vi "GlueRepeatedLinePattern.vi"(2 "Controller In":refnum<k24>, 3 "Dry Run":bool, 5 "Module Number":i32=7, 6 "Calibration Directory":path) -> (0 ".NET Refnum out":refnum<k24>)   [LabVIEW 2016]
uses:
  <vilib>/LabVIEW Interface for Arduino/Type Defs/Arduino Resource.ctl
  <vilib>/LabVIEW Interface for Arduino/Type Defs/Board Type.ctl
  C:/Users/Aerotech/Documents/BNLStaveAssembly-blueprint/Bin/Aerotech.A3200.dll
  BNLStaveAssembly-blueprint/Bin/Aerotech.A3200.dll
  <vilib>/LabVIEW Interface for Arduino/Type Defs/Pin Mode.ctl
  <vilib>/Utility/file.llb/Read Delimited Spreadsheet (DBL).vi
  <vilib>/LabVIEW Interface for Arduino/LabVIEW Interface for Arduino.lvlib
panel:
  out "Line Motion":T1
  out "Finished":bool
  out "N Lines":i32
  out "Lines Glued":i32
  out "Elapsed Time [s]":dbl format="%.2g"
  out "Shift to Start [mm]":dbl[](array[numeric]) format="%.1f"
  out "Start Position [mm]":dbl[](array[numeric]) format="%#.3g"
  in  "Abort stage":bool
  in  "Pattern Indicator":enum32{"Glue Pattern"}(tab)
  out "Relative Line\nSeparations [mm]":dbl[][](array[numeric])=[[18.5, 7.25], [2.5, 3.5], [-3.5, 5.0], [2.5, 3.15], [2.5, 3.15], [2.5, 3.15], [2.5, 3.15], [2.5, 3.15], [2.5, 3.15], [2.5, 3.15], [2.5, 3.15], [2.5, 3.15], [2.5, 3.15], [2.5, 3.15], [3.75, 5.0], [2.5, 3.5]] format="%#_13g"
  out "Line Lengths [mm]":dbl[](array[numeric])=[65.0, 65.0, 73.5, 73.5, 73.5, 73.5, 73.5, 73.5, 73.5, 73.5, 73.5, 73.5, 73.5, 73.5, 65.0, 65.0] format="%#_13g"
  out "Motion Time [s]":dbl[](array[numeric])
  in  "Outputs Tab":enum32{"Running Positions"}(tab)
  out "Running Positions [mm]":dbl[][](array[numeric])
  in  "Times [s]":dbl[](array[numeric])
  out "Running Times [s]":dbl[](array[numeric])
  in  "Inputs Tab":T2(tab)
  out "Virtual Stave Map":path
  out "Stave Angle [rad]":dbl format="%#_13g"
  out "Stereo Angle [mrad]":dbl=-26.0 format="%#_13g"
  out "Total Angle [rad]":dbl
  out "Orientation":string
  out "Pin Down?":bool
  in  "Pulse Length [ms]":dbl=125.0 format="%#_13g"
  out "Arduino Resource":T3={"VISA resource"="GlueCTRL", "Board Type"=enum."Uno", "Connection Type"=enum."USB / Serial", "Bytes Per Packet (15)"=15}
  in  "Digital I/O Pin":u8=7
  in  "Default Axis Speeds":T5={"X [mm/s]"=25.0, "Y [mm/s]"=25.0, "Z [mm/s]"=25.0}
  in  "Camera to Dispenser \nShift [mm]":dbl[](array[numeric])=[107.938, 5.003, 0.0]
  in  "Glue Pattern .csv File":path=path "C:/Users/Aerotech/Documents/BNL_ThermomechanicalStave/1_ModulePlacement/1_GluePatterning/Glue/GluePatterns/Pattern9-8.txt"
  in  "Axial":bool
  in  "Wait [ms]":dbl=750.0 format="%#_13g"
  in  "Positions [mm]":dbl[][](array[numeric])
  in  "Terminate":bool
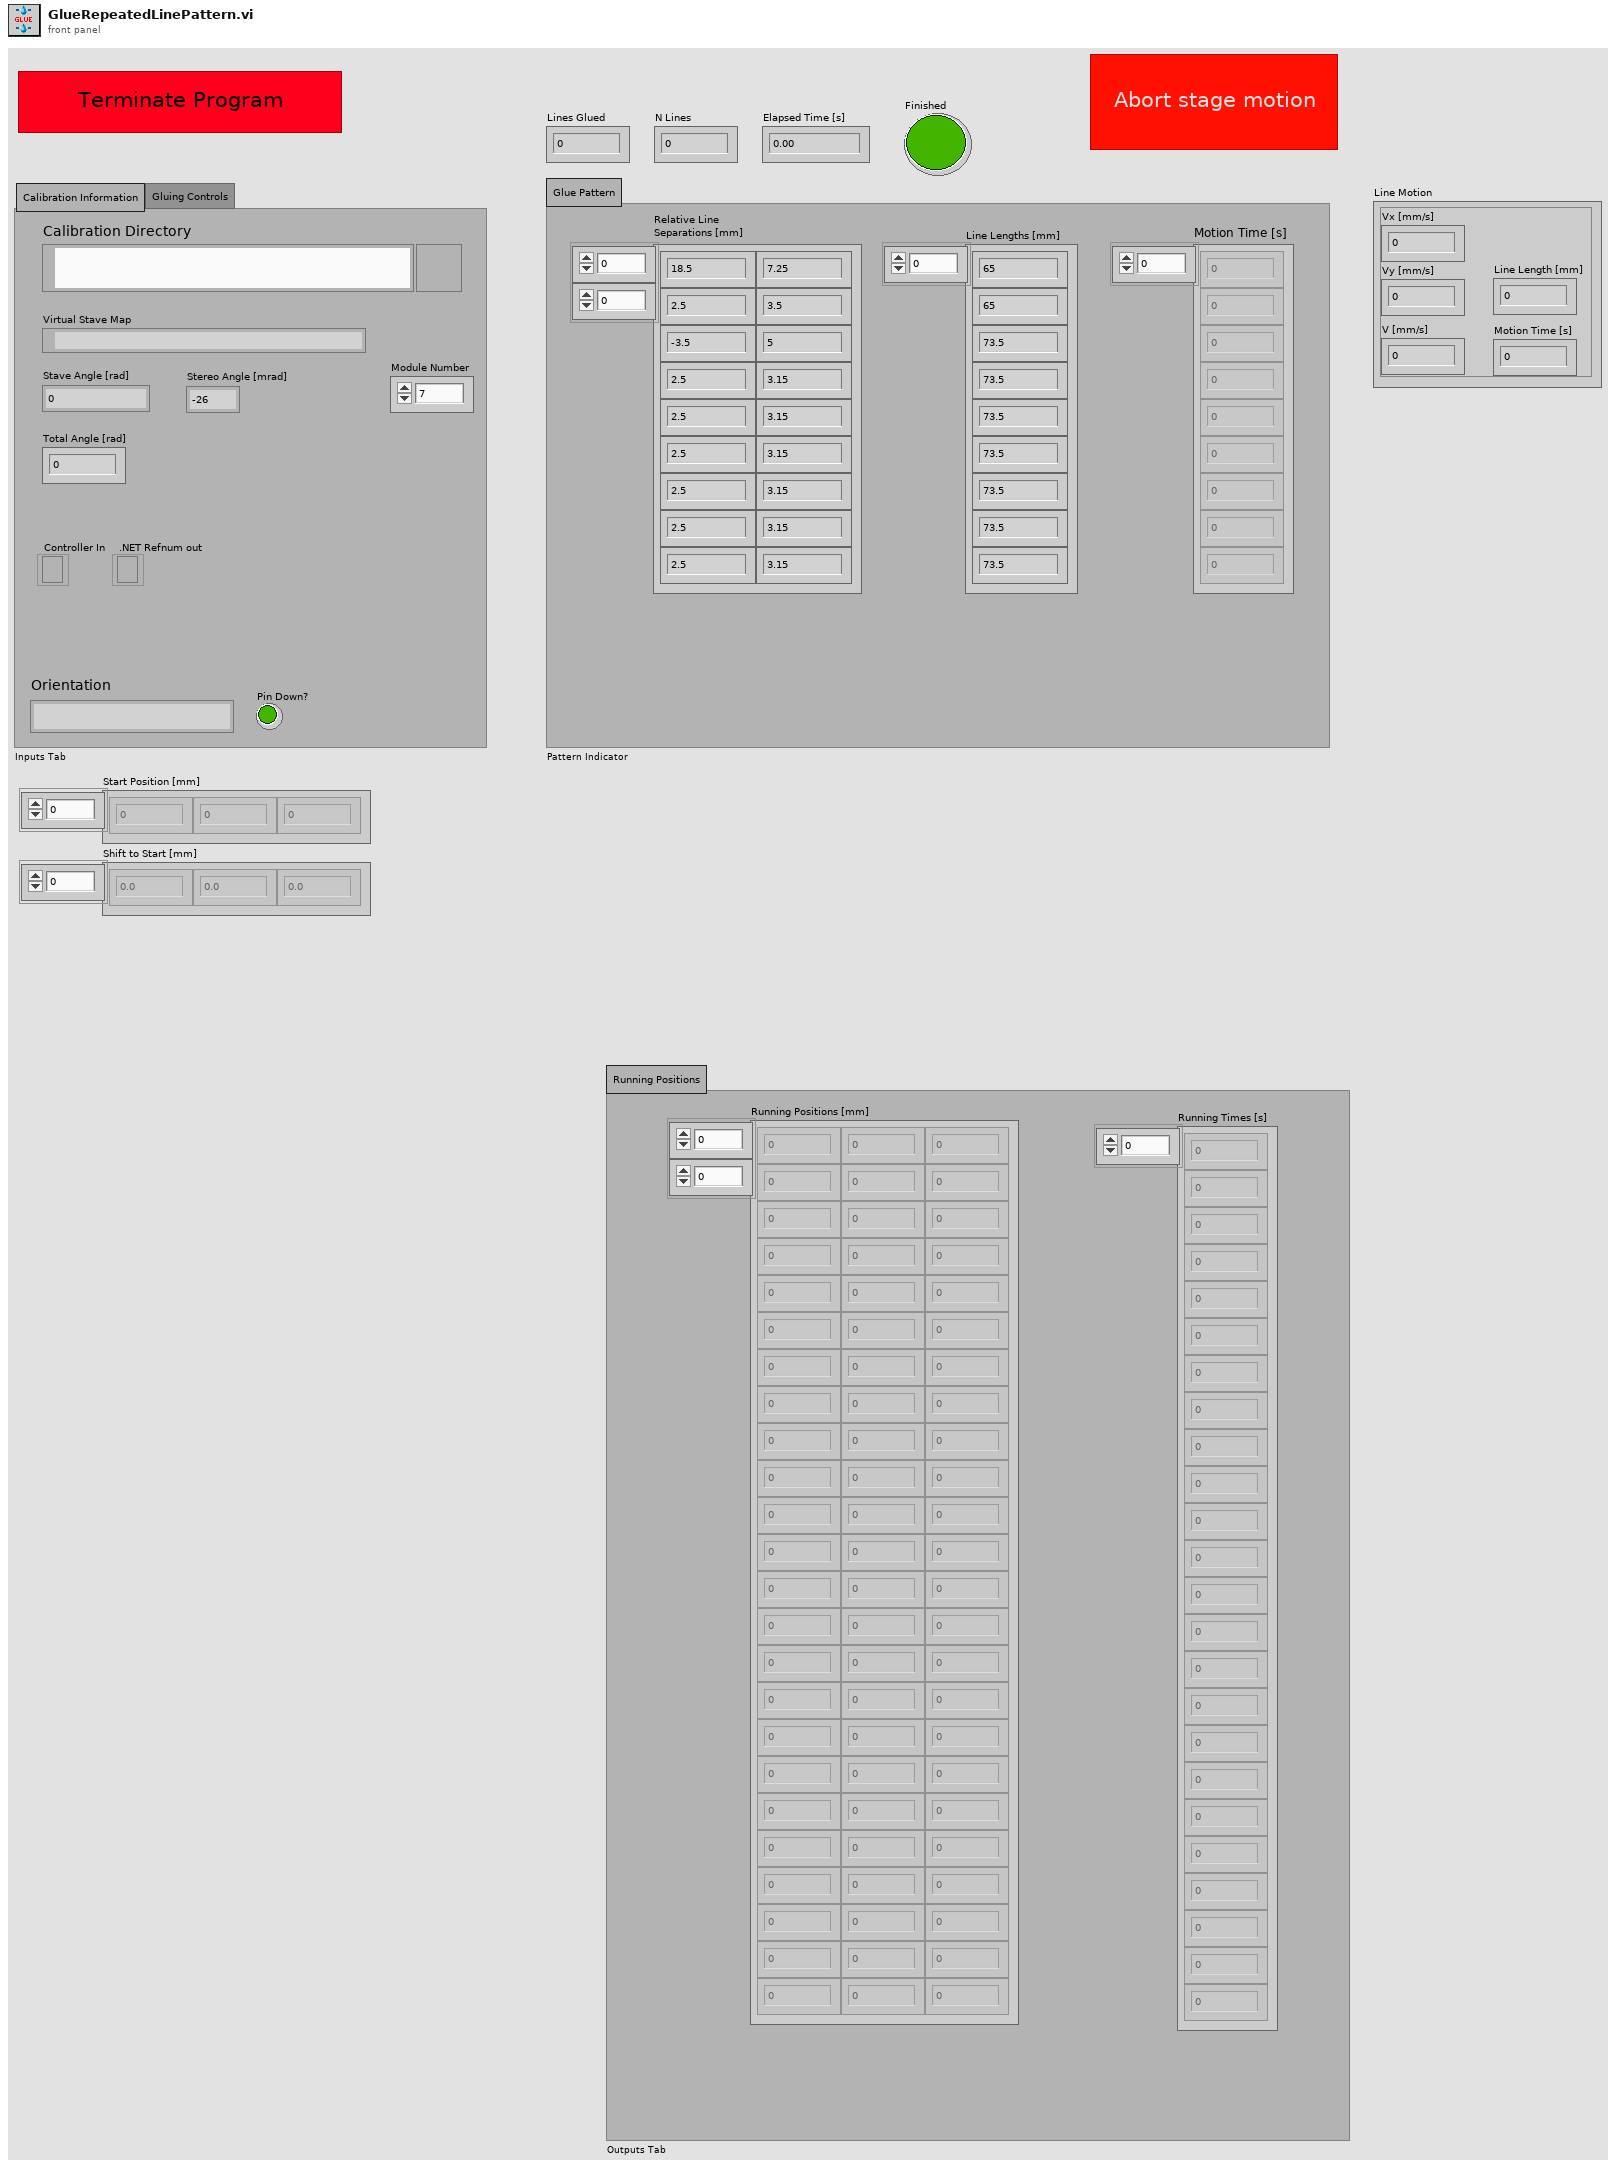
[diagram p1: front panel]
types:
  T1 = cluster{"Vx [mm/s]":dbl, "Vy [mm/s]":dbl, "Numeric Control":dbl, "Numeric Control":dbl, "Line Length [mm]":dbl}
  T2 = enum32{"Calibration Information", "Gluing Controls"}
  T3 = typedef "LabVIEW Interface for Arduino.lvlib/Arduino Resource.ctl" = cluster{"VISA resource":refnum<visa-resource-name>, "Board Type":T4, "Connection Type":enum8{"USB / Serial"}, "Bytes Per Packet (15)":u8}
  T4 = typedef "LabVIEW Interface for Arduino.lvlib/Board Type.ctl" = enum16{"Uno", "Dimuelanove w/Atmega 328", "Mega 2560"}
  T5 = cluster{"X [mm/s]":dbl, "Y [mm/s]":dbl, "Z [mm/s]":dbl}
  T6 = typedef "LabVIEW Interface for Arduino.lvlib/Pin Mode.ctl" = enum8{"Input", "Output"}
  T7 = cluster{"X [mm]":dbl, "Y [mm]":dbl, "Z [mm]":dbl}
  T8 = cluster{"Final X":dbl, "Final Y":dbl, "Final Z":dbl}
  T9 = cluster{"Move to Start of Line [mm][0]":dbl, "Move to Start of Line [mm][1]":dbl, "Move to Start of Line [mm][2]":dbl}
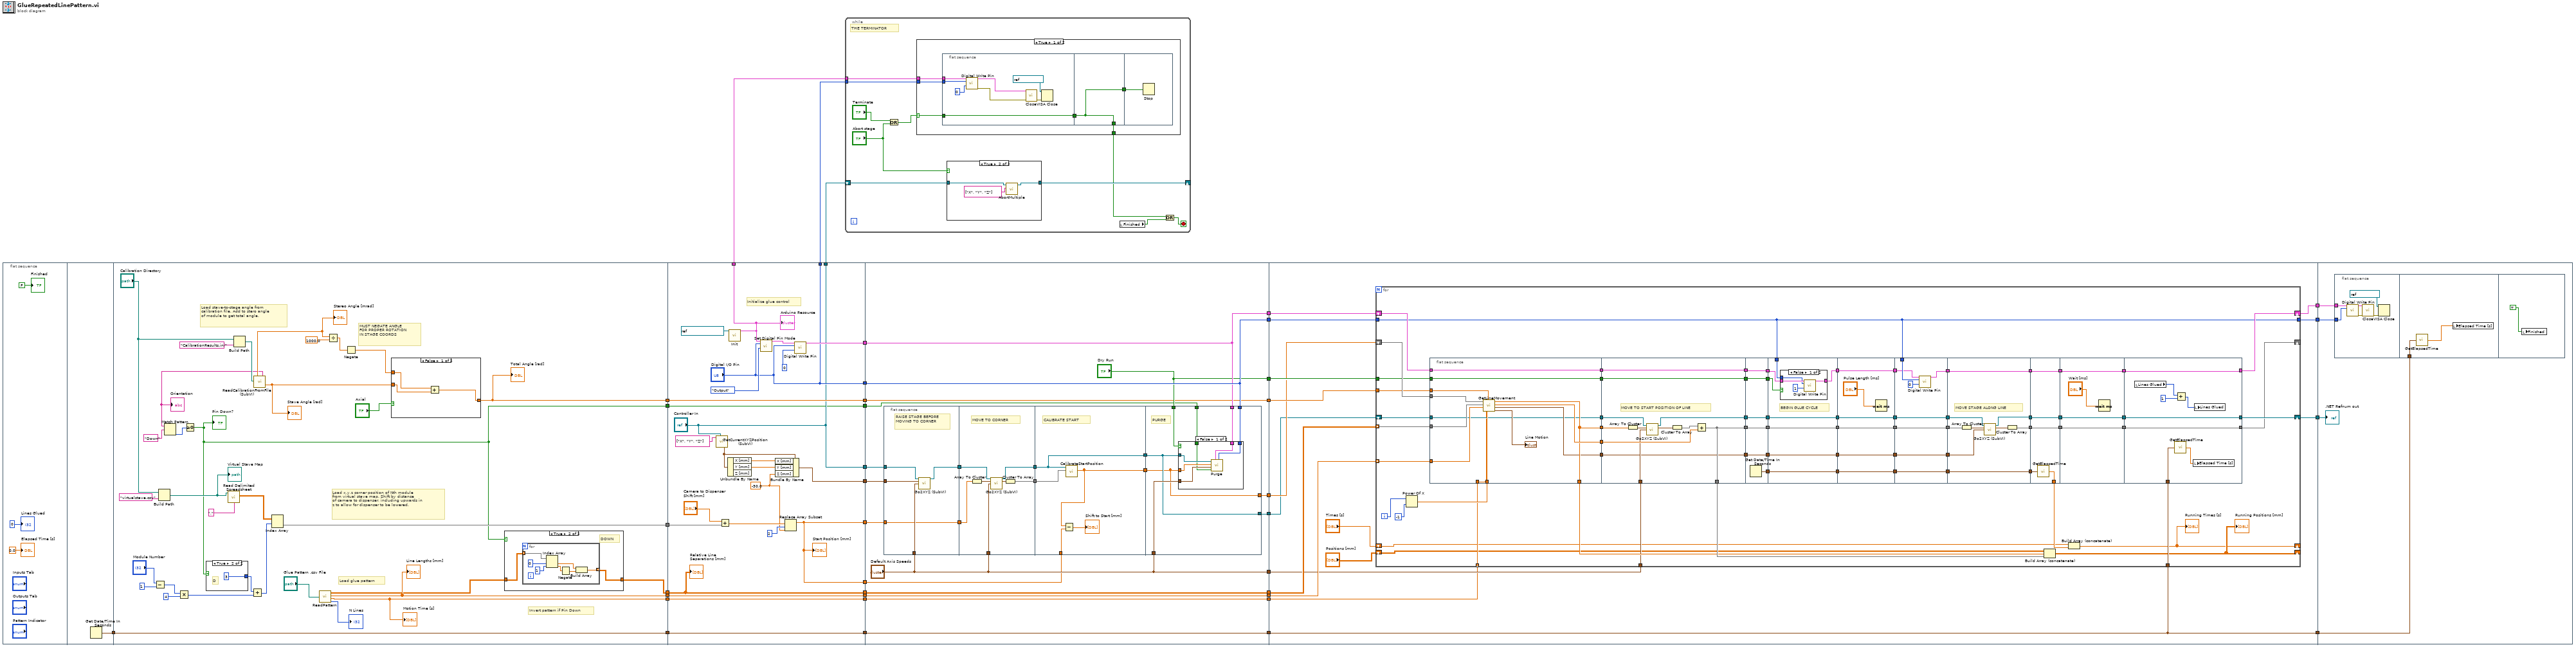
[diagram p0: block diagram]
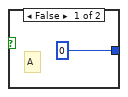
[diagram p2: hidden frame]
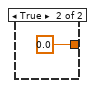
[diagram p3: hidden frame]
diagram:
  n1 = flat-sequence {
    tunnel: [w42] -> w24
    tunnel: [w75] -> w11
    tunnel: [w47] -> w10
    tunnel: [w71] -> w9
    tunnel: [w74] -> w8
    tunnel: [w73] -> w7
    tunnel: [w43] -> w6
    tunnel: [w70] -> w3
    tunnel: w24 -> [w75]
    tunnel: ["Controller In"] -> w38
    tunnel: [w112] -> w37
    tunnel: ["Digital I/O Pin"] -> w36
    tunnel: [w111] -> w30
    tunnel: ["Controller In"] -> w29
    tunnel: [w109] -> w26
    tunnel: w11 -> [w110]
    tunnel: [w110] -> w23
    tunnel: w10 -> [w109]
    tunnel: ["Digital I/O Pin"] -> w20
    tunnel: [w95] -> w17
    tunnel: w9 -> [w95]
    tunnel: w8 -> [w107]
    tunnel: [w107] -> w16
    tunnel: w7 -> [w101]
    tunnel: [w93] -> w14
    tunnel: [w99] -> w13
    tunnel: w6 -> [w94]
    tunnel: [w94] -> w5
    tunnel: [w93] -> w4
    tunnel: w3 -> [w92]
    tunnel: [w92] -> w2
    tunnel: w38 -> [w134]
    tunnel: w37 -> [w132]
    tunnel: w36 -> [w133]
    tunnel: [w133] -> w33
    tunnel: [w132] -> w32
    tunnel: [w131] -> w31
    tunnel: ["Dry Run"] -> w28
    tunnel: [w129] -> w27
    tunnel: w26 -> [w129]
    tunnel: [w128] -> w25
    tunnel: w23 -> [w127]
    tunnel: [w127] -> w22
    tunnel: [w126] -> w19
    tunnel: [w125] -> w18
    tunnel: w17 -> [w126]
    tunnel: w16 -> [w125]
    tunnel: ["Default Axis Speeds"] -> w15
    tunnel: w14 -> [w121]
    tunnel: w13 -> [w120]
    tunnel: w5 -> [w119]
    tunnel: w4 -> [w118]
    tunnel: w2 -> [w117]
    tunnel: [w117] -> w1
    tunnel: [w169] -> w35
    tunnel: [w183] -> w34
    tunnel: w33 -> [w182]
    tunnel: w32 -> [w181]
    tunnel: w31 -> [w177]
    tunnel: w28 -> [w180]
    tunnel: w27 -> [w179]
    tunnel: w25 -> [w178]
    tunnel: w22 -> [w176]
    tunnel: [w176] -> w21
    tunnel: w19 -> [w175]
    tunnel: w18 -> [w174]
    tunnel: w15 -> [w172]
    tunnel: [w171] -> w12
    tunnel: w1 -> [w170]
    tunnel: w35 -> [w338]
    tunnel: w34 -> [w337]
    tunnel: w21 -> [w336]
    tunnel: w12 -> [w335]
    frame #0 {
      "Finished" <- FALSE ("Finished")
      "Elapsed Time [s]" <- 0.0 ("Elapsed Time [s]")
      "Lines Glued" <- 0 ("N Lines")
    }
    frame #1 {
      n2 = Get Date/Time In Seconds() -> (seconds since 1Jan1904=w42:timestamp)
    }
    frame #2 {
      # "Invert pattern if Pin Down"
      # "MUST NEGATE ANGLE \nFOR PROPER ROTATION\nIN STAGE COORDS"
      # "Load glue pattern"
      # "Load x,y,z corner position of Nth module\nfrom virtual stave map. Shift by distance\nof camera to dispenser, including upwards in\nz to allow for dispenser to be lowered."
      # "Load stave-to-stage angle from\ncalibration file. Add to stero angle\nof module to get total angle."
      n3 = Subtract(x="Module Number", y=1) -> (x-y=w60:i32)
      n4 = Build Path(base path="Calibration Directory", name or relative path="virtualstave.csv") -> (appended path=w64:path)
      "Virtual Stave Map" <- w64
      n5 = Multiply(x=w60, y=4) -> (x*y=w54:i32)
      n6 = call-poly <vilib>:"Read Delimited Spreadsheet.vi"("file path (dialog if empty)"=w64, "delimiter (\\t)"="," ("delimiter (\\t)")) -> ("all rows"=w58:dbl[][])  [unwired: 8 in, 5 out]
      n7 = Build Path(base path="Calibration Directory", name or relative path="CalibrationResults.ini") -> (appended path=w66:path)
      n8 = call "ReadCalibrationFromFile (SubVI).vi"("Calibration file path"=w66) -> ("Stereo angle [mrad]"=w48:dbl, "Orientation"=w44:string, "Angle"=w46:dbl)  [unwired: 7 in, 9 out]
      "Stave Angle [rad]" <- w46
      "Stereo Angle [mrad]" <- w48
      "Orientation" <- w44
      n9 = Match Pattern(string=w44, regular expression="Down") -> (offset past match=w51:i32)  [unwired: 1 in, 3 out]
      n10 = Greater Or Equal To 0?(x=w51) -> (x >= 0?=w43:bool)
      "Pin Down?" <- w43
      n11 = case shown="True" w43 {
        tunnel: [0 3] -> w50
        frame False {
          # "A"
        }
        frame True {
          # "D"
        }
      }
      n12 = Add(x=w50, y=w54) -> (x+y=w53:i32)
      n13 = Index Array(array=w58, index (row)=w53) -> (element=w73:dbl[])  [unwired: 1 in]
      n14 = call "ReadPattern.vi"("file path (dialog if empty)"="Glue Pattern .csv File") -> ("Relative Line\nSeparations [mm]"=w72:dbl[][], "Line Lengths [mm]"=w74:dbl[], "Motion Time [s]"=w70:dbl[], "N Lines"=→"N Lines":i32)
      "Line Lengths [mm]" <- w74
      "Motion Time [s]" <- w70
      n15 = Divide(x=w48, y=1000.0) -> (x/y=w49:dbl)
      n16 = Negate(x=w49) -> (-x=w45:dbl)
      n17 = case shown="False" "Axial" {
        tunnel: [w78 0.0] -> w47
        tunnel: w46 -> [w80 _]
        tunnel: w45 -> [w79 _]
        frame False {
          n18 = Add(x=w79, y=w80) -> (x+y=w78:dbl)
        }
        frame True {
        }
      }
      "Total Angle [rad]" <- w47
      n19 = case shown="True" w43 {
        tunnel: w72 -> [w82 w84]
        tunnel: [w82 w83] -> w71
        frame False {
          # "UP"
        }
        frame True {
          # "DOWN"
          n20 = for {
            tunnel: w84 -> [w91] mode=indexing
            tunnel: [w85] -> w83 mode=indexing
            n21 = Index Array(array=w91, index #1=0 ("index"), index #2=1 ("index")) -> (element #1=w87:dbl, element #2=w88:dbl)
            n22 = Negate(x=w88) -> (-x=w86:dbl)
            n23 = Build Array(w87, w86) -> (w85:dbl[])
          }
        }
      }
    }
    frame #3 {
      w96 = -30.0 ("Z [mm]")
      # "Initialize glue control"
      n24 = call "GetCurrentXYZPosition (SubVI).vi"(".NET Refnum in - Device"="Controller In", "Axes Names"=string[] ["X", "Y", "Z"]) -> ("Current stage position"=w104:T7)  [unwired: 4 in, 5 out]
      n25 = Add(x="Camera to Dispenser \nShift [mm]", y=w101) -> (x+y=w98:dbl[])
      n26 = Unbundle By Name(w104) -> ("X [mm]"=w103:dbl, "Y [mm]"=w102:dbl)  [unwired: 1 out]
      n27 = call <vilib>:"Init.vi"("VISA resource"=refnum<visa-resource-name> "GlueCTRL") -> ("Arduino Resource"=w111:T3)  [unwired: 17 in, 1 out]
      "Arduino Resource" <- w111
      n28 = call <vilib>:"Set Digital Pin Mode.vi"("Arduino Resource"=w111, "Digital I/O Pin"="Digital I/O Pin", "Pin Mode (Input)"=Pin_Mode."Output") -> ("Arduino Resource"=w114:T3)  [unwired: 11 in, 1 out]
      n29 = Bundle By Name(cluster=w104, "X [mm]"=w103, "Y [mm]"=w102, "Z [mm]"=w96) -> (w99:T7)
      n30 = Replace Array Subset(array=w98, new element=w96, index=2) -> (w93:dbl[])
      "Start Position [mm]" <- w93
      n31 = call <vilib>:"Digital Write Pin.vi"("Arduino Resource"=w114, "Digital I/O Pin (0)"="Digital I/O Pin", "Value (0)"=u8 0) -> ("Arduino Resource"=w112:T3)  [unwired: 11 in, 1 out]
      "Relative Line\nSeparations [mm]" <- w95
    }
    frame #4 {
      n32 = flat-sequence {
        tunnel: w134 -> [w143]
        tunnel: [w142] -> w124
        tunnel: "Default Axis Speeds" -> [w141]
        tunnel: [w140] -> w122
        tunnel: w121 -> [w140]
        tunnel: w120 -> [w139]
        tunnel: [w147] -> w138
        tunnel: [w146] -> w137
        tunnel: w124 -> [w148]
        tunnel: "Default Axis Speeds" -> [w145]
        tunnel: w122 -> [w144]
        tunnel: w138 -> [w154]
        tunnel: w137 -> [w155]
        tunnel: [w154] -> w136
        tunnel: [w153] -> w135
        tunnel: w118 -> [w152]
        tunnel: w136 -> [w159]
        tunnel: w135 -> [w157]
        tunnel: "Default Axis Speeds" -> [w162]
        tunnel: w133 -> [w161]
        tunnel: w132 -> [w160]
        tunnel: [w159] -> w131
        tunnel: "Dry Run" -> [w158]
        tunnel: [w157] -> w128
        tunnel: w119 -> [w156]
        frame #0 {
          # "RAISE STAGE BEFORE\nMOVING TO CORNER"
          n33 = call "Go2XYZ (SubVI).vi"(".NET Refnum in"=w143, "Go to Coordinates"=w139, "Axis Speeds"=w141) -> (".NET Refnum out"=w142:refnum<k24>)  [unwired: 8 in, 4 out]
        }
        frame #1 {
          # "MOVE TO CORNER"
          n34 = Array To Cluster(array=w144) -> (cluster=w150:cluster{"[0]":dbl, "[1]":dbl, "[2]":dbl})
          n35 = call "Go2XYZ (SubVI).vi"(".NET Refnum in"=w148, "Go to Coordinates"=w150, "Axis Speeds"=w145) -> (".NET Refnum out"=w147:refnum<k24>, "Final Position"=w149:T8)  [unwired: 8 in, 3 out]
          n36 = Cluster To Array(cluster=w149) -> (array=w146:dbl[])
        }
        frame #2 {
          # "CALIBRATE START"
          n37 = call "CalibrateStartPosition.vi"("Start Position [mm]"=w155, ".NET Refnum In"=w154) -> ("Final Position [mm]"=w153:dbl[])  [unwired: 9 in]
          n38 = Subtract(x=w153, y=w152) -> (x-y=→"Shift to Start [mm]":dbl[])
        }
        frame #3 {
          # "PURGE"
          n39 = case shown="False" w158 {
            tunnel: w162 -> [w166 _]
            tunnel: w161 -> [w168 _]
            tunnel: w160 -> [w167 _]
            tunnel: w159 -> [w164 _]
            tunnel: w157 -> [w165 _]
            tunnel: w156 -> [w163 _]
            frame False {
              n40 = call "Purge.vi"("Digital I/O Pin"=w168, "Arduino Resource"=w167, "Pin Down?"=w163, "Axis Speeds"=w166, "Start Position [mm]"=w165, ".NET Refnum In"=w164) -> ()  [unwired: 6 in]
            }
            frame True {
            }
          }
        }
      }
    }
    frame #5 {
      n41 = for {
        tunnel: w175 -> [w213] mode=indexing
        tunnel: w174 -> [w212] mode=indexing
        shift-right: [w245] -> _
        shift-left: w178 -> [w214]
        shift-right: [w246] -> w171
        shift-left: w177 -> [w248]
        shift-right: [w249] -> w169
        shift-left: w181 -> [w247]
        shift-right: [w228] -> _
        shift-left: "Positions [mm]" -> [w186]
        tunnel: w182 -> [w227]
        tunnel: [w227] -> w183
        tunnel: w180 -> [w211]
        tunnel: w179 -> [w210]
        tunnel: w176 -> [w243]
        shift-right: [w187] -> _
        shift-left: "Times [s]" -> [w185]
        tunnel: w172 -> [w189]
        tunnel: w170 -> [w188] mode=indexing
        i -> [w244]
        n42 = Power Of X(1:-1 ("x"), 2:w244) -> (0:w209:dbl)
        n43 = flat-sequence {
          tunnel: [w263] -> w206
          tunnel: [w252] -> w205
          tunnel: [w262] -> w204
          tunnel: [w255] -> w203
          tunnel: [w256] -> w202
          tunnel: [w251] -> _
          tunnel: [w254] -> w195
          tunnel: w247 -> [w263]
          tunnel: w248 -> [w252]
          tunnel: w211 -> [w262]
          tunnel: w214 -> [w260]
          tunnel: w213 -> [w259]
          tunnel: w212 -> [w258]
          tunnel: w210 -> [w261]
          tunnel: w209 -> [w257]
          tunnel: [w255] -> w207
          tunnel: w188 -> [w251]
          tunnel: [w275] -> w242
          tunnel: [w266] -> w241
          tunnel: [w269] -> w240
          tunnel: [w274] -> w239
          tunnel: w206 -> [w275]
          tunnel: w205 -> [w267]
          tunnel: w204 -> [w274]
          tunnel: w203 -> [w268]
          tunnel: w202 -> [w270]
          tunnel: [w269] -> w208
          tunnel: w195 -> [w264]
          tunnel: [w264] -> w192
          tunnel: w189 -> [w265]
          tunnel: w242 -> [w281]
          tunnel: [w281] -> w237
          tunnel: w241 -> [w280]
          tunnel: [w280] -> w236
          tunnel: w240 -> [w279]
          tunnel: [w279] -> w235
          tunnel: w239 -> [w278]
          tunnel: [w278] -> w234
          tunnel: [w277] -> w233
          tunnel: [w276] -> w193
          tunnel: w192 -> [w276]
          tunnel: w237 -> [w286]
          tunnel: w236 -> [w289]
          tunnel: [w289] -> w222
          tunnel: w235 -> [w288]
          tunnel: [w288] -> w220
          tunnel: w234 -> [w284]
          tunnel: w233 -> [w287]
          tunnel: [w287] -> w218
          tunnel: w227 -> [w283]
          tunnel: [w285] -> w216
          tunnel: [w282] -> w194
          tunnel: w193 -> [w282]
          tunnel: w222 -> [w300]
          tunnel: [w300] -> w221
          tunnel: w220 -> [w299]
          tunnel: [w299] -> w219
          tunnel: w218 -> [w298]
          tunnel: [w298] -> w217
          tunnel: w216 -> [w297]
          tunnel: [w297] -> w215
          tunnel: w194 -> [w295]
          tunnel: [w295] -> w190
          tunnel: w221 -> [w308]
          tunnel: [w308] -> w232
          tunnel: w219 -> [w307]
          tunnel: [w307] -> w231
          tunnel: w217 -> [w306]
          tunnel: [w306] -> w230
          tunnel: w215 -> [w303]
          tunnel: [w302] -> w229
          tunnel: w227 -> [w304]
          tunnel: [w301] -> w191
          tunnel: w190 -> [w301]
          tunnel: [w309] -> w226
          tunnel: w232 -> [w310]
          tunnel: w231 -> [w317]
          tunnel: [w316] -> w225
          tunnel: [w315] -> w224
          tunnel: w230 -> [w315]
          tunnel: w229 -> [w314]
          tunnel: [w314] -> w223
          tunnel: w191 -> [w313]
          tunnel: [w318] -> w201
          tunnel: w226 -> [w322]
          tunnel: [w322] -> w199
          tunnel: w225 -> [w321]
          tunnel: [w321] -> w197
          tunnel: w224 -> [w320]
          tunnel: [w319] -> w238
          tunnel: w223 -> [w318]
          tunnel: w201 -> [w326]
          tunnel: [w326] -> w200
          tunnel: w199 -> [w325]
          tunnel: [w325] -> w198
          tunnel: w197 -> [w324]
          tunnel: [w324] -> w196
          tunnel: [w334] -> w249
          tunnel: w200 -> [w334]
          tunnel: [w333] -> w246
          tunnel: w198 -> [w333]
          tunnel: [w332] -> w245
          tunnel: w196 -> [w332]
          tunnel: w243 -> [w328]
          frame #0 {
            n44 = call "GetLineMovement.vi"("Sign"=w257, "Total Angle [rad]"=w261, "Motion Time per Line [s]"=w251, "Line Length [mm]"=w258, "Relative Line\nSeparations [mm]"=w259, "Start Position"=w260) -> ("Line Motion"=→"Line Motion":T1, "Motion Speed [mm/s]"=w254:T5, "Move across Line [mm]"=w256:dbl[], "Move to Start of Line [mm]"=w255:dbl[])
          }
          frame #1 {
            # "MOVE TO START POSITION OF LINE"
            n45 = Array To Cluster(array=w268) -> (cluster=w271:T9)
            n46 = call "Go2XYZ (SubVI).vi"(".NET Refnum in"=w267, "Go to Coordinates"=w271, "Axis Speeds"=w265) -> (".NET Refnum out"=w266:refnum<k24>, "Final Position"=w272:T8)  [unwired: 8 in, 3 out]
            n47 = Cluster To Array(cluster=w272) -> (array=w273:dbl[])
            n48 = Add(x=w273, y=w270) -> (x+y=w269:dbl[])
          }
          frame #2 {
            n49 = Get Date/Time In Seconds() -> (seconds since 1Jan1904=w277:timestamp)
          }
          frame #3 {
            # "BEGIN GLUE CYCLE"
            n50 = case shown="False" w284 {
              tunnel: [w293 w294] -> w285
              tunnel: w286 -> [w292 w294]
              tunnel: w283 -> [w290 _]
              frame False {
                n51 = call <vilib>:"Digital Write Pin.vi"("Arduino Resource"=w292, "Digital I/O Pin (0)"=w290, "Value (0)"=u8 1) -> ("Arduino Resource"=w293:T3)  [unwired: 11 in, 1 out]
              }
              frame True {
              }
            }
          }
          frame #4 {
            n52 = Wait (ms)(milliseconds to wait="Pulse Length [ms]") -> ()  [unwired: 1 out]
          }
          frame #5 {
            n53 = call <vilib>:"Digital Write Pin.vi"("Arduino Resource"=w303, "Digital I/O Pin (0)"=w304, "Value (0)"=u8 0) -> ("Arduino Resource"=w302:T3)  [unwired: 11 in, 1 out]
          }
          frame #6 {
            # "MOVE STAGE ALONG LINE"
            n54 = Array To Cluster(array=w317) -> (cluster=w311:cluster{"[0]":dbl, "[1]":dbl, "[2]":dbl})
            n55 = call "Go2XYZ (SubVI).vi"(".NET Refnum in"=w310, "Go to Coordinates"=w311, "Axis Speeds"=w313) -> (".NET Refnum out"=w309:refnum<k24>, "Final Position"=w312:T8)  [unwired: 8 in, 3 out]
            n56 = Cluster To Array(cluster=w312) -> (array=w316:dbl[])
          }
          frame #7 {
            n57 = call "GetElapsedTime.vi"("Start Time"=w320) -> ("Elapsed Time [s]"=w319:sgl)
          }
          frame #8 {
            n58 = Wait (ms)(milliseconds to wait="Wait [ms]") -> ()  [unwired: 1 out]
          }
          frame #9 {
            n59 = local read "Lines Glued"() -> (w330:i32)
            n60 = call "GetElapsedTime.vi"("Start Time"=w328) -> ("Elapsed Time [s]"=w327:sgl)
            n61 = Add(x=w330, y=1) -> (x+y=w331:i32)
            n62 = local write "Elapsed Time [s]"(w327) -> ()
            n63 = local write "Lines Glued"(w331) -> ()
          }
        }
        n64 = Build Array (concatenate)(w186, w207, w208) -> (w228:dbl[][])
        "Running Positions [mm]" <- w228
        n65 = Build Array (concatenate)(w185, w238) -> (w187:dbl[])
        "Running Times [s]" <- w187
      }
    }
    frame #6 {
      n66 = flat-sequence {
        tunnel: w338 -> [w340]
        tunnel: w337 -> [w339]
        tunnel: w336 -> [w345]
        frame #0 {
          n67 = call <vilib>:"Digital Write Pin.vi"("Arduino Resource"=w340, "Digital I/O Pin (0)"=w339) -> ("Arduino Resource"=w343:T3, "error out"=w342:errorcluster)  [unwired: 12 in]
          n68 = call <vilib>:"Close.vi"("Arduino Resource"=w343, "error in"=w342) -> ("error out"=w341:errorcluster)  [unwired: 13 in]
          n69 = VISA Close(VISA resource name=refnum<visa-resource-name> "GlueCTRL", error in (no error)=w341) -> ()  [unwired: 1 out]
        }
        frame #1 {
          n70 = call "GetElapsedTime.vi"("Start Time"=w345) -> ("Elapsed Time [s]"=w346:sgl)
          n71 = local write "Elapsed Time [s]"(w346) -> ()
        }
        frame #2 {
          n72 = local write "Finished"(TRUE ("stop? (T)")) -> ()
        }
      }
      ".NET Refnum out" <- w335
    }
  }
  n73 = while {
    tunnel: w30 -> [w357]
    shift-right: [w355] -> _
    shift-left: w29 -> [w356]
    tunnel: w20 -> [w349]
    stop <- w352 stop-if-true
    # "THE TERMINATOR"
    n74 = Or(x="Terminate", y="Abort stage") -> (x .or. y?=w351:bool)
    n75 = case shown="True" w351 {
      selector: w351 -> [w367 w378]
      tunnel: w357 -> [w365 _]
      tunnel: [w363 w378] -> w350
      tunnel: w349 -> [w362 _]
      frame True {
        n76 = flat-sequence {
          tunnel: [w373] -> w366
          tunnel: w362 -> [w369]
          tunnel: w365 -> [w371]
          tunnel: w367 -> [w373]
          tunnel: w366 -> [w376]
          tunnel: [w376] -> w364
          tunnel: [w376] -> w363
          tunnel: w364 -> [w377]
          frame #0 {
            n77 = call <vilib>:"Digital Write Pin.vi"("Arduino Resource"=w371, "Digital I/O Pin (0)"=w369, "Value (0)"=u8 0) -> ("Arduino Resource"=w372:T3, "error out"=w368:errorcluster)  [unwired: 11 in]
            n78 = call <vilib>:"Close.vi"("Arduino Resource"=w372, "error in"=w368) -> ("error out"=w374:errorcluster)  [unwired: 13 in]
            n79 = VISA Close(VISA resource name=refnum<visa-resource-name> "GlueCTRL", error in (no error)=w374) -> ()  [unwired: 1 out]
          }
          frame #1 {
          }
          frame #2 {
            n80 = Stop(stop? (T)=w377) -> ()
          }
        }
      }
      frame False {
      }
    }
    n81 = case shown="True" "Abort stage" {
      tunnel: w356 -> [w358 w360]
      tunnel: [w358 w359] -> w355
      frame False {
      }
      frame True {
        n82 = call "AbortMultiple.vi"("axis names"=string[] ["X", "Y", "Z"], "controller in"=w360) -> ("controller out"=w359:refnum<k24>)  [unwired: 8 in, 1 out]
      }
    }
    n83 = local read "Finished"() -> (w348:bool)
    n84 = Or(x=w350, y=w348) -> (x .or. y?=w352:bool)
  }
